vi "Register Test.vi"(8 "error in (no error)":errorcluster, 10 "VI Call Chain":string[](array[string]), 11 "Assert Factory in":refnum<class "Test Assert Factory.lvclass">) -> (0 "error out":errorcluster, 3 "Assert Factory out":refnum<class "Test Assert Factory.lvclass">)   [LabVIEW 2013, in "Caraya.lvlib" / "Test Assert Factory.lvclass"]
doc: "Registers a Test VI with the Assert Factory"
uses:
  Test Assert Factory.lvclass
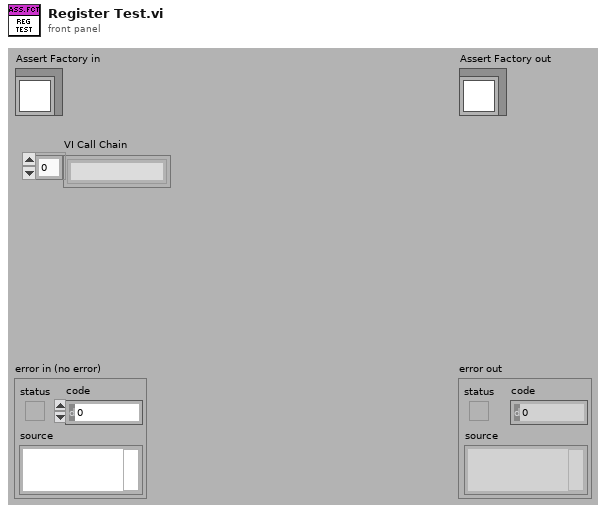
[diagram p1: front panel]
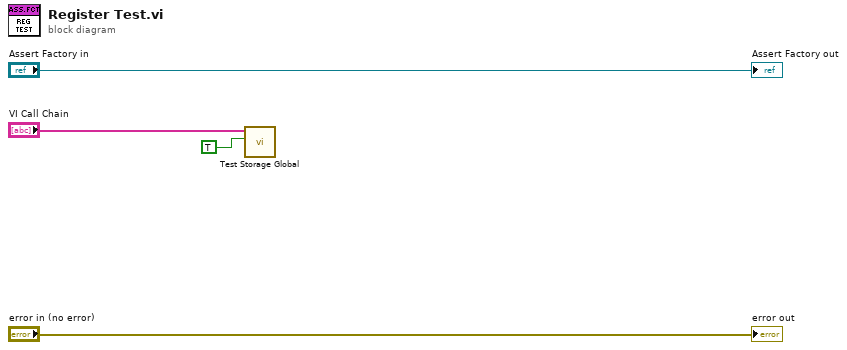
[diagram p0: block diagram]
diagram:
  n1 = call "Test Storage Global.vi"("Set (F)"=TRUE, "VI Call Chain"="VI Call Chain") -> ()  [unwired: 8 in, 2 out]
  "error out" <- "error in (no error)"
  "Assert Factory out" <- "Assert Factory in"
